vi "New Image (ARGB Array).vi"(7 "Set Alpha Values to 255 (Default: True)":bool=TRUE, 8 "error in (no error)":errorcluster, 11 "U32 ARBG Data  (Default: Empty)":u32[][](array[numeric])) -> (0 "error out":errorcluster, 3 "New ARGB Image":T1)   [LabVIEW 2020, in "g_ar_toolkit.image.lvlib"]
uses:
  g_ar_toolkit.image.lvlib
  ARGB Image.ctl
  g_ar_toolkit.common/g_ar_toolkit.common.lvlib
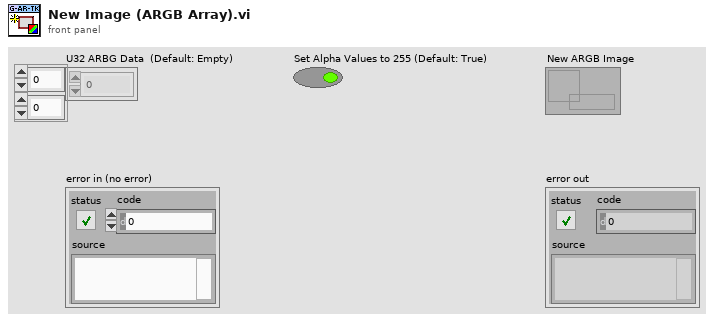
[diagram p1: front panel]
types:
  T1 = typedef "g_ar_toolkit.image.lvlib/ARGB Image.ctl" = refnum<data-value>
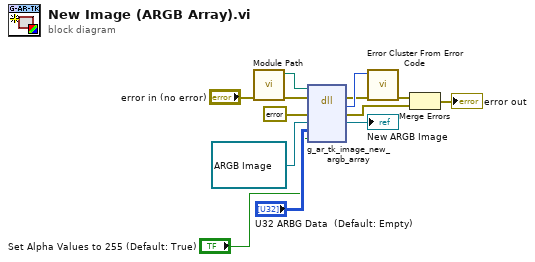
[diagram p0: block diagram]
diagram:
  n1 = call "Module Path.vi"("error in (no error)"="error in (no error)") -> ("error out"=w5:errorcluster, "Path"=w4:path)  [unwired: 9 in]
  n2 = dll-call lib="?" fn="g_ar_tk_image_new_argb_array" ("g_ar_toolkit.*.*:g_ar_tk_image_create")(path in=w4, error in=w5, "error_cluster"=errorcluster {"status"=FALSE, "code"=0, "source"=""} ("error constant"), "EDVR"=T1 refnum ("ARGB Image"), "array_handle"="U32 ARBG Data  (Default: Empty)", "set_alpha_channel_to_255"="Set Alpha Values to 255 (Default: True)") -> (error out=w6:errorcluster, "MgErr"=w7:i32, "error_cluster"=w13:errorcluster, "EDVR"=→"New ARGB Image":T1)  [unwired: 3 in, 1 out]
  n3 = call <vilib>:"Error Cluster From Error Code.vi"("error in (no error)"=w6, "error code (0)"=w7) -> ("error out"=w9:errorcluster)  [unwired: 7 in]
  n4 = Merge Errors(w9, w13) -> (→"error out":errorcluster)
